vi "Store Static VI References for Subpanel.vi"(8 "error in (no error)":errorcluster, 11 "DAQ Configuration in":refnum<class "DAQ Configuration.lvclass">) -> (0 "error out":errorcluster, 3 "DAQ Configuration out":refnum<class "DAQ Configuration.lvclass">)   [LabVIEW 2017, in "Hardware.lvlib" / "DAQ Configuration.lvclass"]
uses:
  DAQ Configuration.lvclass
  C:/Program Files (x86)/National Instruments/LabVIEW 2017/user.lib/Configuration Dialog Actor/Configuration.lvclass
  MAL-Framework/user.lib/Common Components/Hardware/HW Config/HW Configuration.vi
  MAL-Framework/user.lib/Common Components/Hardware/HW with output config.lvclass
  <userlib>/Configuration Dialog Actor/Configuration.lvclass
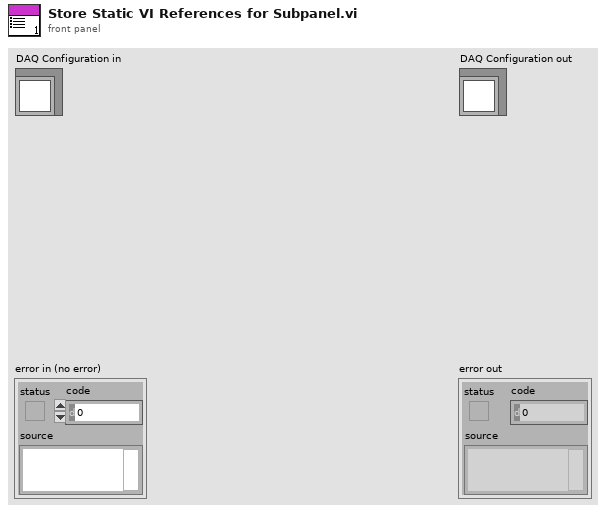
[diagram p1: front panel]
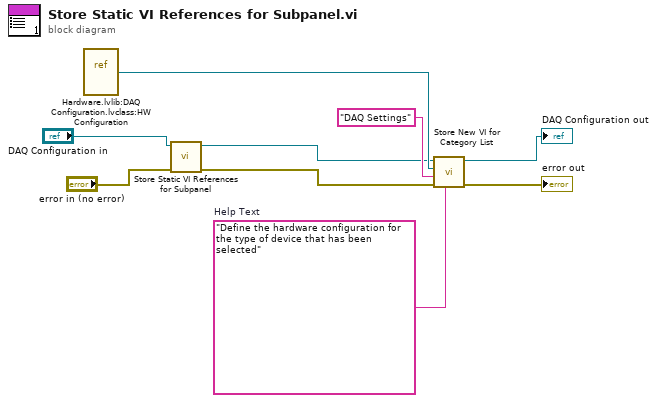
[diagram p0: block diagram]
diagram:
  w6 = "Define the hardware configuration for the type of device that has been selected"  # Help Text
  n1 = vi-ref "Hardware.lvlib:DAQ Configuration.lvclass:HW Configuration.vi"() -> (w7:refnum<vi>)
  n2 = call-parent "Store Static VI References for Subpanel.vi"("error in (no error)"="error in (no error)", "HW with output config in"="DAQ Configuration in") -> ("error out"=w2:errorcluster, "HW with output config out"=w3:refnum<class "DAQ Configuration.lvclass">)  [unwired: 8 in]
  n3 = call <userlib>:"Store New VI for Category List.vi"("Help Text"=w6, "error in (no error)"=w2, "String"="DAQ Settings", "VI Refnum"=w7, "Configuration in"=w3) -> ("error out"=→"error out":errorcluster, "Configuration out"=→"DAQ Configuration out":refnum<class "DAQ Configuration.lvclass">)  [unwired: 5 in]
